vi "CloneClass.vi"(0 "ClassWriterNative.lvclass":refnum<class "ClassWriterNative.lvclass">, 1 "ClassRef":refnum<vi>, 2 "NewClassPath":path, 5 "error in (no error)":errorcluster) -> (14 "ClassWriterNative.lvclass":refnum<class "ClassWriterNative.lvclass">, 16 "NewClassPathOut(Might Be Modified)":path, 19 "error out":errorcluster)   [LabVIEW 2014, in "ClassWriterNative.lvclass"]
uses:
  <resource>/Framework/Providers/Open_GDS/ClassProviders/Provider_LvNativeClass/ClassWriterNative_class/ClassWriterNative.lvclass
  <vilib>/Utility/miscctls.llb/LVPointTypeDef.ctl
  <resource>/Framework/Providers/Open_GDS/ClassProviders/Common/ScriptingFunctions/Scripting.lvclass
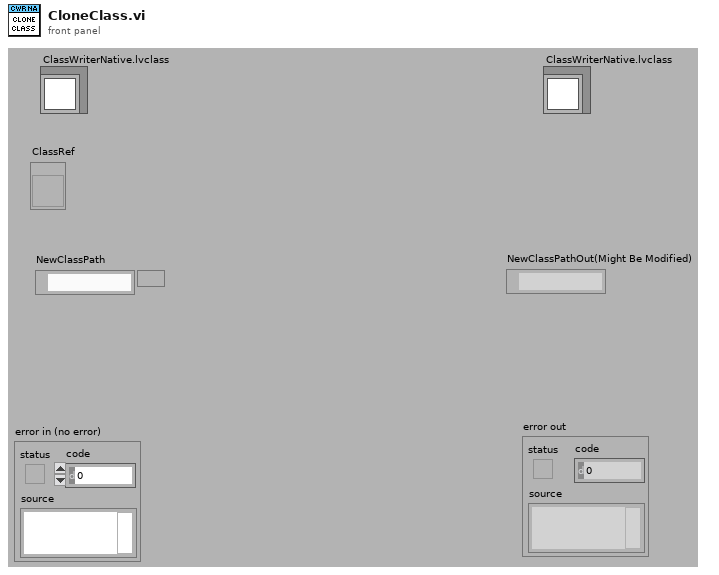
[diagram p1: front panel]
types:
  T1 = cluster{"NewClass":refnum<vi>, "OrgClassName":string, "NewClassName":string, "ProjectItemToAddTo":refnum<vi>, "Path":path, "Application":refnum<vi>, "VIRefs":refnum<vi>[]}
  T2 = typedef "LVPointTypeDef.ctl" = cluster{"Horizontal":i16, "Vertical":i16}
  T3 = enum32{"not a control VI", "control", "typedef", "strict typedef"}
  T4 = enum32{"invalid VI type", "Standard VI", "Control VI", "Global VI", "Polymorphic VI", "Configuration VI", "SubSystem", "Facade VI", "Method VI", "Statechart Diagram VI"}
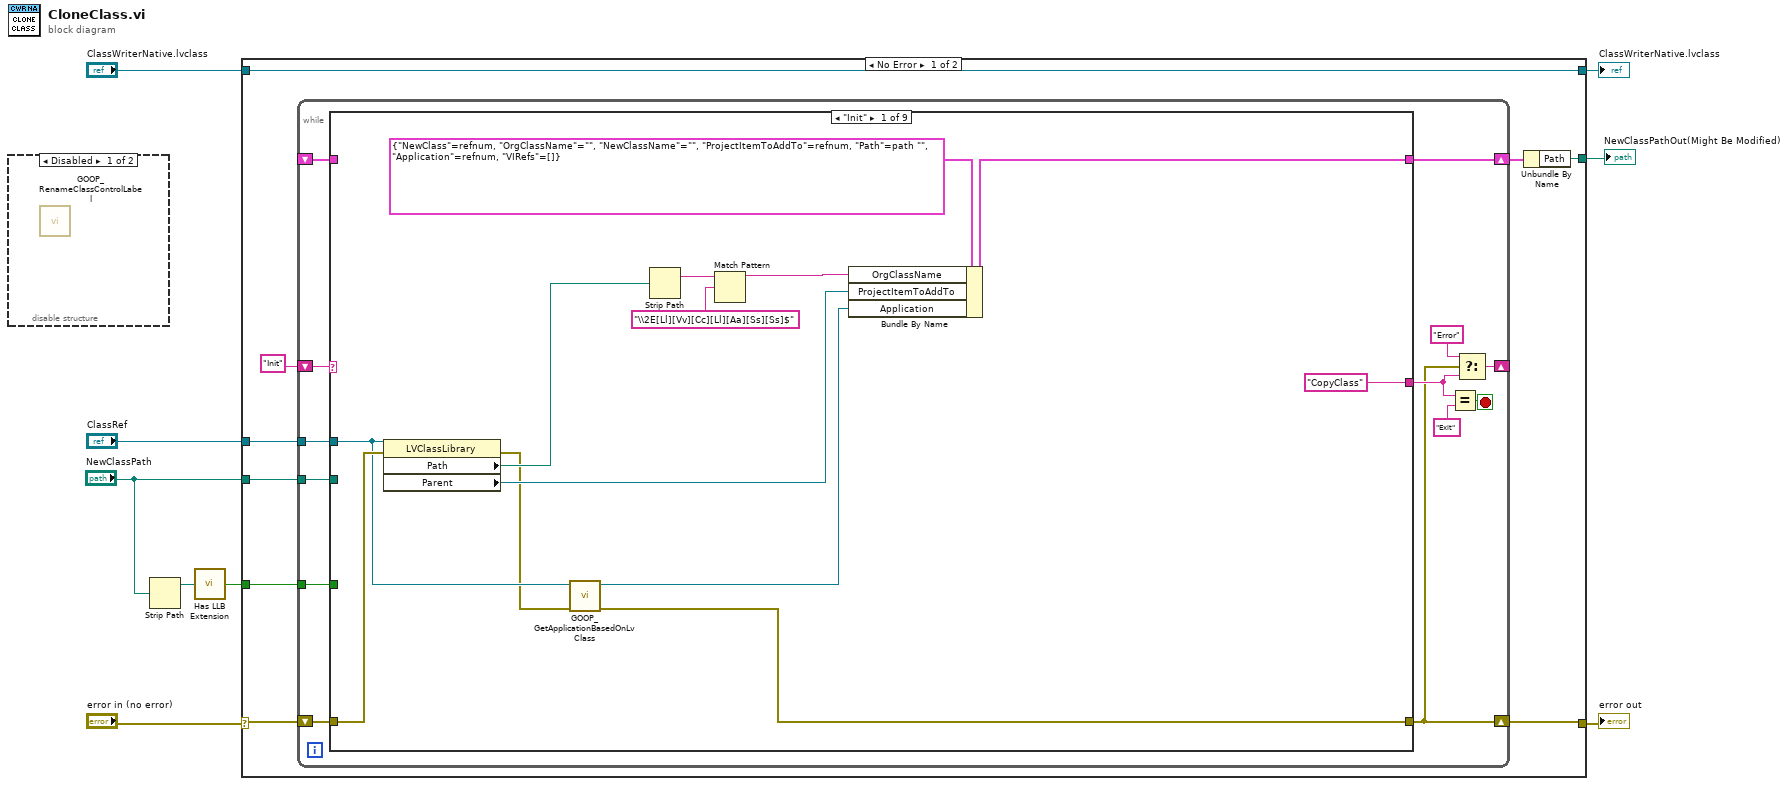
[diagram p0: block diagram]
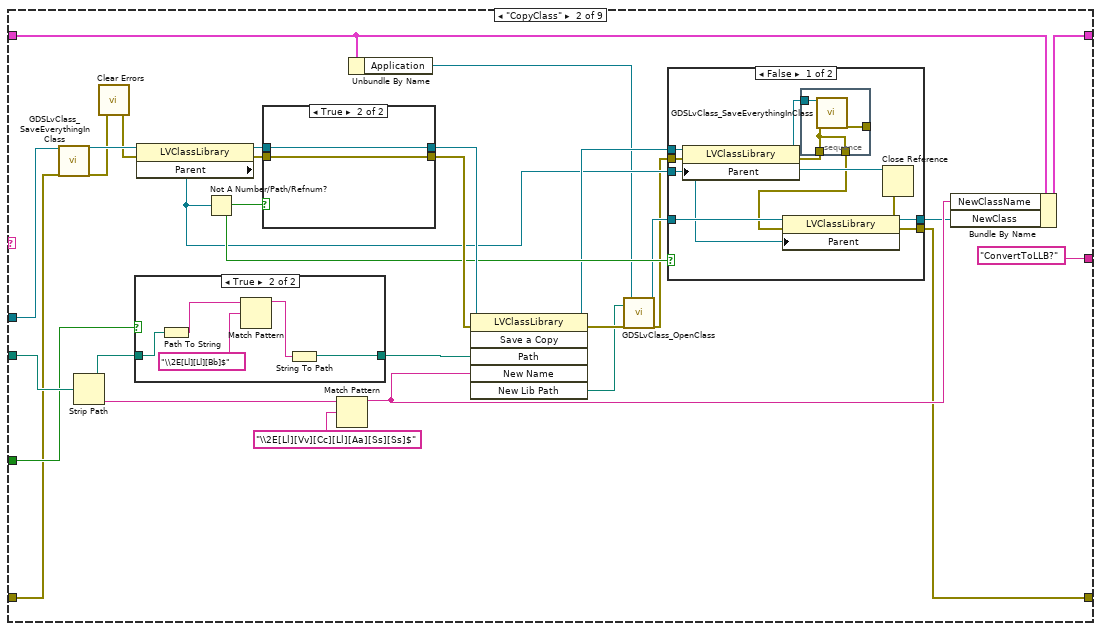
[diagram p3: hidden frame]
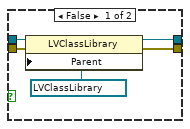
[diagram p6: hidden frame]
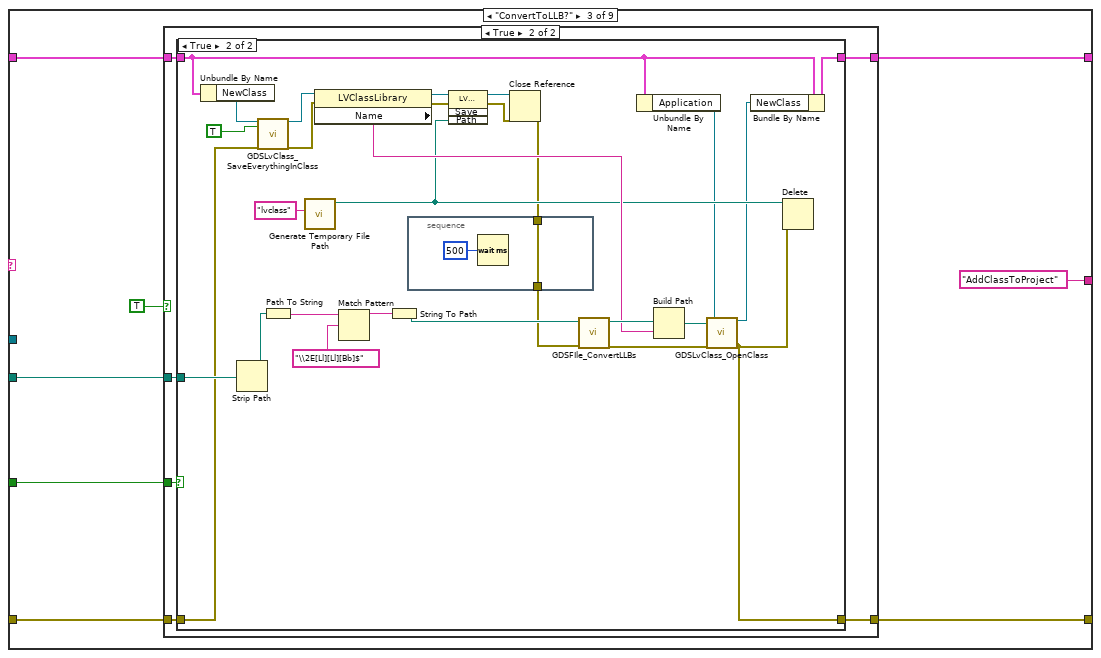
[diagram p7: hidden frame]
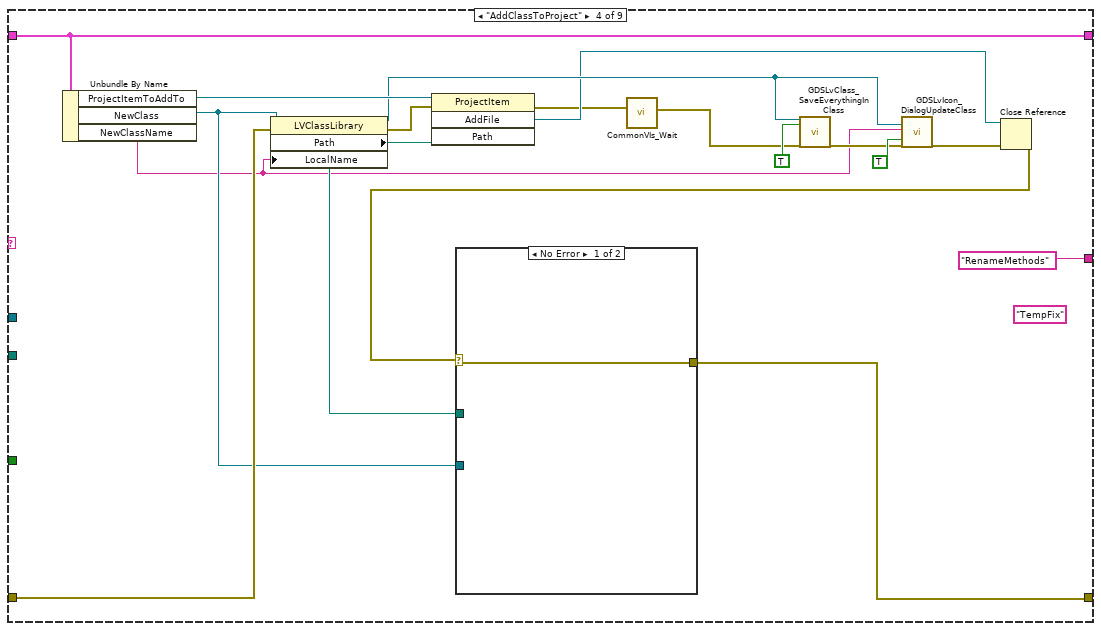
[diagram p10: hidden frame]
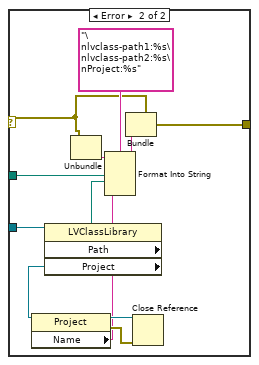
[diagram p11: hidden frame]
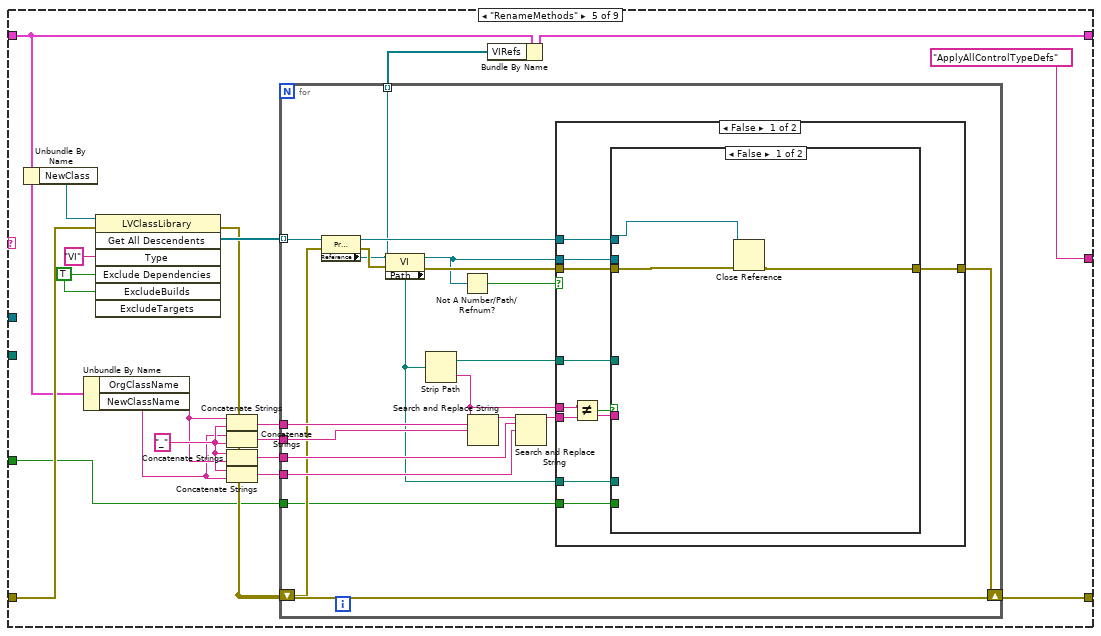
[diagram p12: hidden frame]
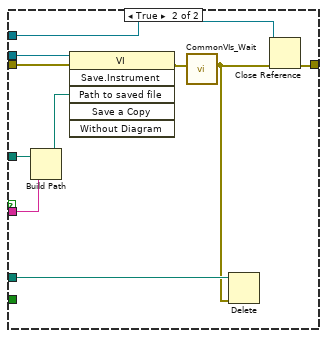
[diagram p13: hidden frame]
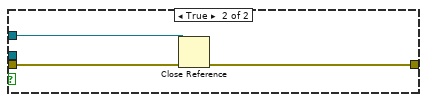
[diagram p14: hidden frame]
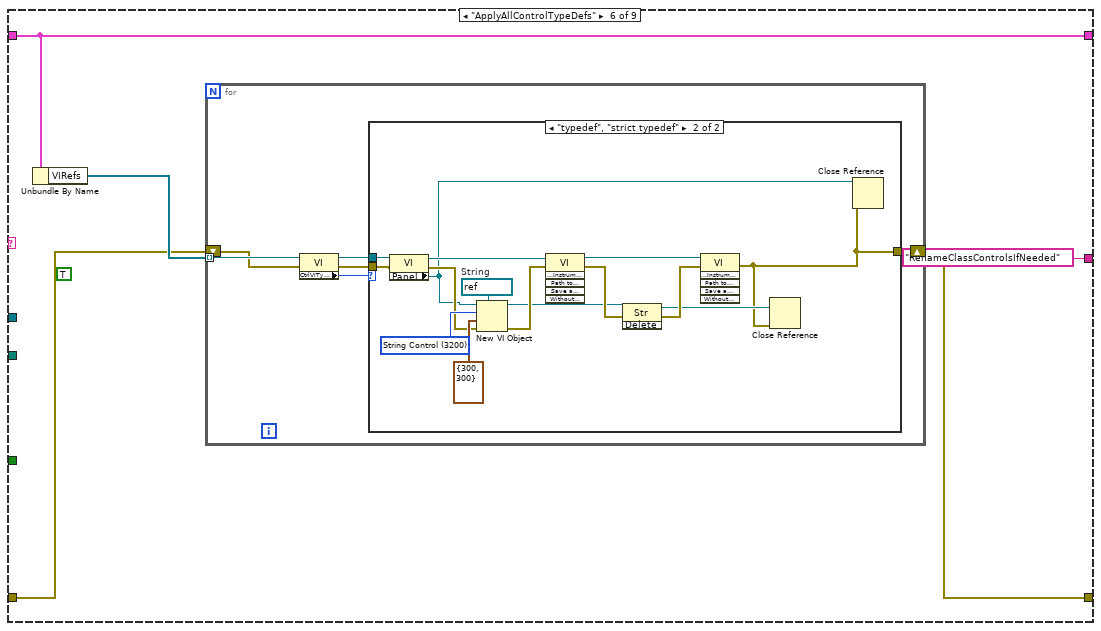
[diagram p15: hidden frame]
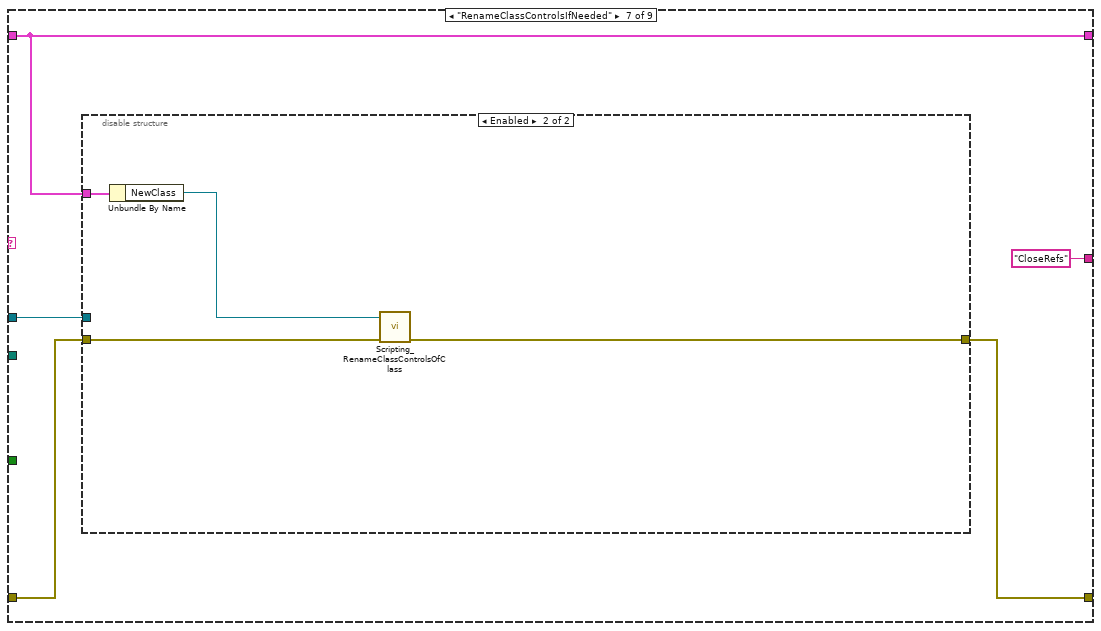
[diagram p17: hidden frame]
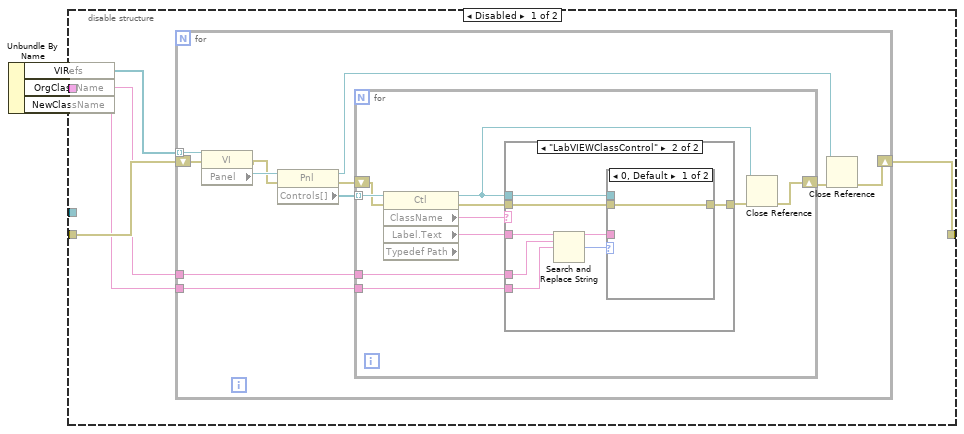
[diagram p18: hidden frame]
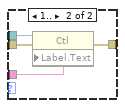
[diagram p20: hidden frame]
diagram:
  n1 = disable-structure shown="Disabled" {
    frame Disabled {
      n2 = call <resource>:"GOOP_RenameClassControlLabel.vi"() -> ()  [unwired: 10 in, 2 out]
    }
    frame Enabled {
    }
  }
  n3 = Strip Path(path="NewClassPath") -> (stripped path=w4:path)  [unwired: 1 out]
  n4 = call <vilib>:"Has LLB Extension.vi"("path"=w4) -> ("path to VI library?"=w2:bool)
  n5 = case shown="No Error" "error in (no error)" {
    selector: "error in (no error)" -> [w16 w385]
    tunnel: [w15 w385] -> w8
    tunnel: "ClassWriterNative.lvclass" -> [w18 w384]
    tunnel: [w18 w384] -> w6
    tunnel: "ClassRef" -> [w14 _]
    tunnel: "NewClassPath" -> [w13 _]
    tunnel: w2 -> [w12 _]
    tunnel: [w10 _] -> w1
    frame No Error {
      n6 = while {
        shift-right: [w24] -> w15
        shift-left: w16 -> [w31]
        shift-right: [w29] -> _
        shift-left: "Init" -> [w30]
        shift-right: [w23] -> w11
        shift-left: _ -> [w22]
        tunnel: w14 -> [w21]
        tunnel: w13 -> [w20]
        tunnel: w12 -> [w19]
        stop <- w28 stop-if-true
        n7 = case shown="\"Init\"" w30 {
          tunnel: w31 -> [w40 w49 w105 w162 w189 w243 w272 w321 w346]
          tunnel: [w32 w54 w104 w153 w186 w246 w273 w323 w345] -> w24
          tunnel: ["CopyClass" "ConvertToLLB?" "AddClassToProject" "RenameMethods" "ApplyAllControlTypeDefs" "RenameClassControlsIfNeeded" "CloseRefs" "Exit" "CloseRefs"] -> w25
          tunnel: [w38 w71 w101 w164 w181 w247 w274 w327 w347] -> w23
          tunnel: w22 -> [_ w46 w102 w164 w185 w247 w274 w328 w347]
          tunnel: w21 -> [w35 w67 _ _ _ _ w270 _ _]
          tunnel: w20 -> [_ w69 w107 _ _ _ _ _ _]
          tunnel: w19 -> [_ w50 w106 _ w183 _ _ _ _]
          frame "Init" {
            n8 = property class="LVClassLibrary"(reference=w35, error in=w40) -> (error out=w33:errorcluster, "Path"=w41:path, "Parent"=w36:refnum<vi>)  [unwired: 1 out]
            n9 = call <resource>:"GOOP_GetApplicationBasedOnLvClass.vi"("error in (no error)"=w33, "LVClassLibrary in"=w35) -> ("error out"=w32:errorcluster, "Application out"=w34:refnum<vi>)  [unwired: 8 in]
            n10 = Strip Path(path=w41) -> (name=w43:string)  [unwired: 1 out]
            n11 = Match Pattern(string=w43, regular expression="\\2E[Ll][Vv][Cc][Ll][Aa][Ss][Ss]$") -> (before substring=w37:string)  [unwired: 1 in, 3 out]
            n12 = Bundle By Name(cluster=T1 {"NewClass"=refnum, "OrgClassName"="", "NewClassName"="", "ProjectItemToAddTo"=refnum, "Path"=path "", "Application"=refnum, "VIRefs"=[]}, "OrgClassName"=w37, "ProjectItemToAddTo"=w36, "Application"=w34) -> (w38:T1)
          }
          frame "CopyClass" {
            n13 = call <resource>:"GDSLvClass_SaveEverythingInClass.vi"("ClassRefIn"=w67, "error in"=w49) -> ("ClassRefOut"=w64:refnum<vi>, "error out"=w48:errorcluster)  [unwired: 16 in]
            n14 = Strip Path(path=w69) -> (stripped path=w51:path, name=w73:string)
            n15 = call <vilib>:"Clear Errors.vi"("error in (no error)"=w48) -> ("error out"=w47:errorcluster)  [unwired: 5 in, 1 out]
            n16 = case shown="True" w50 {
              tunnel: w51 -> [w74 w79]
              tunnel: [w74 w78] -> w53
              frame False {
              }
              frame True {
                n17 = Path To String(path=w79) -> (string=w77:string)
                n18 = Match Pattern(string=w77, regular expression="\\2E[Ll][Ll][Bb]$") -> (before substring=w75:string)  [unwired: 1 in, 3 out]
                n19 = String To Path(string=w75) -> (path=w78:path)
              }
            }
            n20 = property class="LVClassLibrary"(reference=w64, error in=w47) -> (reference out=w66:refnum<vi>, error out=w63:errorcluster, "Parent"=w58:refnum<vi>)
            n21 = Not A Number/Path/Refnum?(number/path/refnum=w58) -> (NaN/Path/Refnum?=w60:bool)
            n22 = case shown="True" w60 {
              tunnel: w66 -> [w98 w100]
              tunnel: w63 -> [w96 w99]
              tunnel: [w95 w99] -> w62
              tunnel: [w94 w100] -> w61
              frame False {
                n23 = property class="LVClassLibrary"(reference=w98, error in=w96, "Parent"=refnum<vi> refnum ("Parent Class")) -> (reference out=w94:refnum<vi>, error out=w95:errorcluster)
              }
              frame True {
              }
            }
            n24 = Match Pattern(string=w73, regular expression="\\2E[Ll][Vv][Cc][Ll][Aa][Ss][Ss]$") -> (before substring=w65:string)  [unwired: 1 in, 3 out]
            n25 = Unbundle By Name(w46) -> ("Application"=w45:refnum<vi>)
            n26 = invoke class="LVClassLibrary" method="Save a Copy"(reference=w61, error in=w62, "Path"=w53, "New Name"=w65) -> (reference out=w59:refnum<vi>, error out=w70:errorcluster, "New Lib Path"=w68:path)  [unwired: 2 in, 3 out]
            n27 = call <resource>:"GDSLvClass_OpenClass.vi"("ClassToOpen"=w68, "error in (no error)"=w70, "Project/ApplicationRef(If empty, currect active project will be used)"=w45) -> ("LVClass.Open"=w57:refnum<vi>, "error out"=w55:errorcluster)  [unwired: 15 in]
            n28 = case shown="False" w60 {
              tunnel: w59 -> [w88 _]
              tunnel: w55 -> [w87 w92]
              tunnel: w58 -> [w83 _]
              tunnel: w57 -> [w86 w93]
              tunnel: [w85 w93] -> w56
              tunnel: [w84 w92] -> w54
              frame False {
                n29 = property class="LVClassLibrary"(reference=w88, error in=w87, "Parent"=w83) -> (reference out=w82:refnum<vi>, error out=w81:errorcluster)
                n30 = stacked-sequence {
                  tunnel: w82 -> [w91]
                  tunnel: w81 -> [w90]
                  tunnel: [w90] -> w80
                  tunnel: [w89] -> _
                  frame #0 {
                    n31 = call <resource>:"GDSLvClass_SaveEverythingInClass.vi"("ClassRefIn"=w91, "error in"=w90) -> ("error out"=w89:errorcluster)  [unwired: 16 in, 1 out]
                  }
                }
                n32 = property class="LVClassLibrary"(reference=w86, error in=w80, "Parent"=w83) -> (reference out=w85:refnum<vi>, error out=w84:errorcluster)
                n33 = Close Reference(reference=w83, error in (no error)=w84) -> ()  [unwired: 1 out]
              }
              frame True {
              }
            }
            n34 = Bundle By Name(cluster=w46, "NewClassName"=w65, "NewClass"=w56) -> (w71:T1)
          }
          frame "ConvertToLLB?" {
            n35 = case shown="True" TRUE {
              tunnel: w107 -> [_ w116]
              tunnel: w106 -> [_ w115]
              tunnel: w105 -> [w110 w114]
              tunnel: [w110 w113] -> w104
              tunnel: w102 -> [w109 w112]
              tunnel: [w109 w111] -> w101
              frame False {
              }
              frame True {
                n36 = case shown="True" w115 {
                  tunnel: w116 -> [_ w143]
                  tunnel: w114 -> [w118 w134]
                  tunnel: [w118 w123] -> w113
                  tunnel: w112 -> [w117 w122]
                  tunnel: [w117 w140] -> w111
                  frame False {
                  }
                  frame True {
                    n37 = Unbundle By Name(w122) -> ("NewClass"=w136:refnum<vi>)
                    n38 = Strip Path(path=w143) -> (stripped path=w142:path)  [unwired: 1 out]
                    n39 = call <resource>:"GDSLvClass_SaveEverythingInClass.vi"("ClassRefIn"=w136, "ForceResaving(False)"=TRUE, "error in"=w134) -> ("ClassRefOut"=w135:refnum<vi>, "error out"=w133:errorcluster)  [unwired: 15 in]
                    n40 = Path To String(path=w142) -> (string=w146:string)
                    n41 = call <vilib>:"Generate Temporary File Path.vi"("Temporary File Extension (tmp)"="lvclass") -> ("Unique Temporary File Path"=w127:path)  [unwired: 9 in, 1 out]
                    n42 = property class="LVClassLibrary"(reference=w135, error in=w133) -> (reference out=w130:refnum<vi>, error out=w129:errorcluster, "Name"=w138:string)
                    n43 = Match Pattern(string=w146, regular expression="\\2E[Ll][Ll][Bb]$") -> (before substring=w144:string)  [unwired: 1 in, 3 out]
                    n44 = String To Path(string=w144) -> (path=w141:path)
                    n45 = invoke class="LVClassLibrary" method="Save"(reference=w130, error in=w129, "Path"=w127) -> (reference out=w125:refnum<vi>, error out=w124:errorcluster)  [unwired: 1 in, 2 out]
                    n46 = Close Reference(reference=w125, error in (no error)=w124) -> (error out=w120:errorcluster)
                    n47 = stacked-sequence {
                      tunnel: w120 -> [w148]
                      tunnel: [w148] -> w119
                      frame #0 {
                        n48 = Wait (ms)(milliseconds to wait=u32 500) -> ()  [unwired: 1 out]
                      }
                    }
                    n49 = call <resource>:"GDSFIle_ConvertLLBs.vi"("error in (no error)"=w119, "ClassPath Or LLB Path"=w141) -> ("error out"=w132:errorcluster, "ClassPath Or LLB Path Out"=w139:path)  [unwired: 8 in]
                    n50 = Unbundle By Name(w122) -> ("Application"=w121:refnum<vi>)
                    n51 = Build Path(base path=w139, name or relative path=w138) -> (appended path=w131:path)
                    n52 = call <resource>:"GDSLvClass_OpenClass.vi"("ClassToOpen"=w131, "error in (no error)"=w132, "Project/ApplicationRef(If empty, currect active project will be used)"=w121) -> ("LVClass.Open"=w126:refnum<vi>, "error out"=w123:errorcluster)  [unwired: 15 in]
                    n53 = Bundle By Name(cluster=w122, "NewClass"=w126) -> (w140:T1)
                    n54 = Delete(path (use dialog)=w127, error in=w123) -> ()  [unwired: 3 in, 3 out]
                  }
                }
              }
            }
          }
          frame "AddClassToProject" {
            (unwired) "TempFix"
            n55 = Unbundle By Name(w164) -> ("ProjectItemToAddTo"=w166:refnum<vi>, "NewClass"=w158:refnum<vi>, "NewClassName"=w149:string)
            n56 = property class="LVClassLibrary"(reference=w158, error in=w162, "LocalName"=w149) -> (reference out=w160:refnum<vi>, error out=w165:errorcluster, "Path"=w157:path)
            n57 = invoke class="ProjectItem" method="AddFile"(reference=w166, error in=w165, "Path"=w157) -> (error out=w151:errorcluster, "AddFile"=w156:refnum<vi>)  [unwired: 1 in, 2 out]
            n58 = call <resource>:"CommonVIs_Wait.vi"("error in"=w151) -> ("error out"=w150:errorcluster)  [unwired: 9 in]
            n59 = call <resource>:"GDSLvClass_SaveEverythingInClass.vi"("ClassRefIn"=w160, "ForceResaving(False)"=TRUE, "error in"=w150) -> ("error out"=w159:errorcluster)  [unwired: 15 in, 1 out]
            n60 = call <resource>:"GDSLvIcon_DialogUpdateClass.vi"("ClassPath(FilePath/ProjectTreePath/LvCLassRef)"=w160, "ClassName"=w149, "AutoUpdate"=TRUE, "error in (no error)"=w159) -> ("error out"=w155:errorcluster)  [unwired: 12 in, 3 out]
            n61 = Close Reference(reference=w156, error in (no error)=w155) -> (error out=w154:errorcluster)
            n62 = case shown="No Error" w154 {
              selector: w154 -> [w167 w168]
              tunnel: w158 -> [_ w173]
              tunnel: w157 -> [_ w172]
              tunnel: [w167 w171] -> w153
              frame No Error {
              }
              frame Error {
                n63 = property class="LVClassLibrary"(reference=w173) -> ("Path"=w178:path, "Project"=w177:refnum<vi>)  [unwired: 1 in, 2 out]
                n64 = property class="Project"(reference=w177) -> (reference out=w176:refnum<vi>, error out=w175:errorcluster, "Name"=w174:string)  [unwired: 1 in]
                n65 = Unbundle(w168) -> ("source"=w170:string)  [unwired: 2 out]
                n66 = Format Into String(format string="\nlvclass-path1:%s\nlvclass-path2:%s\nProject:%s", initial string=w170, w172, w178, w174) -> (resulting string=w169:string)  [unwired: 1 in, 1 out]
                n67 = Bundle(cluster=w168, "source"=w169) -> (w171:errorcluster)  [unwired: 2 in]
                n68 = Close Reference(reference=w176, error in (no error)=w175) -> ()  [unwired: 1 out]
              }
            }
          }
          frame "RenameMethods" {
            w184 = TRUE ("ExcludeDependencies")
            w193 = "_" ("string")
            n69 = Unbundle By Name(w185) -> ("NewClass"=w197:refnum<vi>)
            n70 = Unbundle By Name(w185) -> ("OrgClassName"=w188:string, "NewClassName"=w187:string)
            n71 = invoke class="LVClassLibrary" method="Get All Descendents"(reference=w197, error in=w189, "Type"="VI", "Exclude Dependencies"=w184, "ExcludeBuilds"=w184) -> (error out=w186:errorcluster, "All Descendents"=w190:refnum<vi>[])  [unwired: 2 in, 5 out]
            n72 = Concatenate Strings(w188, w193) -> (w192:string)
            n73 = Concatenate Strings(w187, w193) -> (w191:string)
            n74 = Concatenate Strings(w193, w188) -> (w194:string)
            n75 = Concatenate Strings(w193, w187) -> (w195:string)
            n76 = for {
              tunnel: w190 -> [w205] mode=indexing
              tunnel: w192 -> [w216]
              tunnel: w191 -> [w215]
              tunnel: w194 -> [w212]
              tunnel: w195 -> [w211]
              shift-right: [w201] -> _
              shift-left: w186 -> [w210]
              tunnel: w183 -> [w199]
              tunnel: [w198] -> w180 mode=indexing
              n77 = property class="ProjectItem"(reference=w205, error in=w210) -> (reference out=w204:refnum<vi>, error out=w209:errorcluster, "Reference"=w198:refnum<vi>)
              n78 = property class="VI"(reference=w198, error in=w209) -> (reference out=w200:refnum<vi>, error out=w202:errorcluster, "Path"=w203:path)
              n79 = Strip Path(path=w203) -> (stripped path=w206:path, name=w207:string)
              n80 = Not A Number/Path/Refnum?(number/path/refnum=w200) -> (NaN/Path/Refnum?=w214:bool)
              n81 = Search and Replace String(input string=w207, search string=w216, replace string=w215) -> (result string=w213:string)  [unwired: 5 in, 3 out]
              n82 = Search and Replace String(input string=w213, search string=w212, replace string=w211) -> (result string=w208:string)  [unwired: 5 in, 3 out]
              n83 = case shown="False" w214 {
                tunnel: w200 -> [w226 _]
                tunnel: w208 -> [w223 _]
                tunnel: w207 -> [w225 _]
                tunnel: w206 -> [w222 _]
                tunnel: w204 -> [w221 w242]
                tunnel: w203 -> [w220 _]
                tunnel: w202 -> [w219 w241]
                tunnel: [w218 w240] -> w201
                tunnel: w199 -> [w217 _]
                frame False {
                  n84 = Not Equal?(x=w225, y=w223) -> (x != y?=w224:bool)
                  n85 = case shown="False" w224 {
                    tunnel: w226 -> [_ w236]
                    tunnel: w223 -> [_ w239]
                    tunnel: w222 -> [_ w238]
                    tunnel: w221 -> [w228 w233]
                    tunnel: w220 -> [_ w235]
                    tunnel: w219 -> [w227 w234]
                    tunnel: [w229 w232] -> w218
                    tunnel: w217 -> [_ _]
                    frame False {
                      n86 = Close Reference(reference=w228, error in (no error)=w227) -> (error out=w229:errorcluster)
                    }
                    frame True {
                      n87 = Build Path(base path=w238, name or relative path=w239) -> (appended path=w237:path)
                      n88 = invoke class="VI" method="Save.Instrument"(reference=w236, error in=w234, "Path to saved file"=w237) -> (error out=w231:errorcluster)  [unwired: 3 in, 5 out]
                      n89 = call <resource>:"CommonVIs_Wait.vi"("error in"=w231) -> ("error out"=w230:errorcluster)  [unwired: 9 in]
                      n90 = Delete(path (use dialog)=w235, error in=w230) -> ()  [unwired: 3 in, 3 out]
                      n91 = Close Reference(reference=w233, error in (no error)=w230) -> (error out=w232:errorcluster)
                    }
                  }
                }
                frame True {
                  n92 = Close Reference(reference=w242, error in (no error)=w241) -> (error out=w240:errorcluster)
                }
              }
            }
            n93 = Bundle By Name(cluster=w185, "VIRefs"=w180) -> (w181:T1)
          }
          frame "ApplyAllControlTypeDefs" {
            (unwired) TRUE ("ExcludeDependencies")
            n94 = Unbundle By Name(w247) -> ("VIRefs"=w244:refnum<vi>[])
            n95 = for {
              shift-right: [w252] -> w246
              shift-left: w243 -> [w248]
              tunnel: w244 -> [w249] mode=indexing
              n96 = property class="VI"(reference=w249, error in=w248) -> (reference out=w251:refnum<vi>, error out=w253:errorcluster, "CtrlVIType"=w250:T3)
              n97 = case shown="\"typedef\", \"strict typedef\"" w250 {
                tunnel: w251 -> [_ w267]
                tunnel: w253 -> [w254 w264]
                tunnel: [w254 w255] -> w252
                frame Default {
                }
                frame "typedef", "strict typedef" {
                  w268 = refnum<vi> refnum  # String
                  w269 = 3200 items=[".NET Refnum"=3441, "Absolute Value"=1054, "Access Rights"=1412, "ActiveX Container"=2072, "Add"=1050, "Add Array Elements"=1903, "Agitator"=3831, "AllSpoll"=1960, "And"=1061, "And Array Elements"=1911, "Append True/False String"=1511, "Application Refnum"=3412, "Array"=3300, "Array 1"=21608, "Array Constant"=2070, "Array Max & Min"=1907, "Array Size"=1809, "Array Subset"=2044, "Array To Cluster"=1168, "Array To Spreadsheet String"=1540, "Array of Strings to Path"=1422, "Atmospheric Tank"=3070, "Atmospheric Tank 1"=21751, "Automation Close"=8001, "Automation Open"=8000, "Automation Refnum"=3410, "Avogadro Constant (1/mol)"=2030, "Base 10 Logarithm Of e"=2022, "Bin"=3073, "Bin 1"=21755, "Boolean Array To Number"=1815, "Boolean To (0,1)"=1167, "Build Array"=2041, "Build Cluster Array"=2047, "Build Path"=1419, "Build Waveform"=2066, "Bundle"=2049, "Bundle By Name"=2057, "Byte Array To String"=1609, "Byte Stream File Refnum"=3408, "Call By Reference Node"=3901, "Call Chain"=1999, "Call Library Function Node"=2062, "Cancel Button"=3131, "Cancel Button 1"=21739, "Cancel Notification"=9107, "Carriage Return Constant"=2010, "Case Structure"=2001, "Cast Unit Bases"=1079, "Check Valve"=3833, "Checkbox"=3117, "Class Specifier Constant"=2094, "Close File"=1405, "Close Reference"=8011, "Cluster"=3400, "Cluster 1"=21607, "Cluster Constant"=2071, "Cluster To Array"=1169, "Code Interface Node"=2050, "Color Box"=3013, "Color Box Constant"=2120, "Color Box Thin Border"=2905, "Color Ramp"=3022, "Combo Box"=21604, "Combo Box 1"=3304, "Combo Box Constant"=2088, "Complex Conjugate"=1048, "Complex To Polar"=1045, "Complex To Re/Im"=1044, "Compound Arithmetic"=2200, "Compressor"=3832, "Concatenate Strings"=2040, "Conditional Disable Structure"=2064, "Constructor Node"=3904, "Control Help Window"=1353, "Control Online Help"=1355, "Control Refnum"=3419, "Convert Unit"=2059, "Conveyer"=3827, "Copy"=1416, "Cosecant"=1204, "Cosine"=1201, "Cotangent"=1205, "Create User Event"=2073, "Current VI's Menubar"=9000, "Current VI's Path"=1426, "DAQmx Analog Trigger Source"=3336, "DAQmx Analog Trigger Source 1"=21774, "DAQmx Analog Trigger Source 2"=21951, "DAQmx Analog Trigger Source Constant"=2119, "DAQmx Device Name"=3318, "DAQmx Device Name 1"=21950, "DAQmx Device Name 2"=21773, "DAQmx Device Name Constant"=2093, "DAQmx Global Channel"=3443, "DAQmx Global Channel 1"=21770, "DAQmx Global Channel 2"=21957, "DAQmx Global Channel Constant"=3430, "DAQmx Physical Channel"=21777, "DAQmx Physical Channel 1"=21954, "DAQmx Physical Channel 2"=3335, "DAQmx Physical Channel Constant"=2118, "DAQmx Scale Name"=21952, "DAQmx Scale Name 1"=21775, "DAQmx Scale Name 2"=3317, "DAQmx Scale Name Constant"=2116, "DAQmx Switch"=21953, "DAQmx Switch 1"=3337, "DAQmx Switch 2"=21776, "DAQmx Switch Constant"=2121, "DAQmx Task Name"=3442, "DAQmx Task Name 1"=21778, "DAQmx Task Name 2"=21959, "DAQmx Task Name Constant"=3434, "DAQmx Terminal"=21955, "DAQmx Terminal 1"=21781, "DAQmx Terminal 2"=3319, "DAQmx Terminal Constant"=2117, "Data Log File Refnum"=3402, "DataSocket Close"=1085, "DataSocket Open"=1084, "DataSocket Read"=1086, "DataSocket Refnum"=3417, "DataSocket Write"=1087, "Database Variant To Data"=8004, "Date/Time To Seconds"=1308, "Decimal Digit?"=1119, "Decimal String To Number"=1184, "Decimate 1D Array"=2046, "Decrement"=1058, "Default Directory"=1427, "Delete"=1417, "Delete From Array"=3912, "Delete Menu Items"=9004, "Delete Variant Attribute"=8206, "Delete Waveform Attribute"=8209, "Dequeue Element"=9113, "Destroy User Event"=2075, "DevClear"=1961, "DevClearList"=1962, "Device Control/Status"=1433, "Device Refnum"=3405, "Diagram Disable Structure"=2054, "Dial"=21732, "Dial 1"=3050, "Dialog Button"=3130, "Dialog Checkbox"=3132, "Dialog Chiseled Line"=3632, "Dialog Colored Rectangle"=3625, "Dialog Combo Box"=21917, "Dialog Horizontal Pointer Slide"=21902, "Dialog Horizontal Progress Bar"=21910, "Dialog Horizontal Slide"=21904, "Dialog Label"=21961, "Dialog Listbox"=2105, "Dialog Listbox 1"=21921, "Dialog Multicolumn Listbox"=21220, "Dialog Multiple Selection Multicolumn Listbox"=21221, "Dialog Numeric"=21919, "Dialog Path Control"=21922, "Dialog Pict Ring"=21925, "Dialog Radio Button"=3133, "Dialog Recessed Frame"=3624, "Dialog Ring"=3060, "Dialog Spin Control"=21900, "Dialog String"=21920, "Dialog Tab Control"=3331, "Dialog Table"=21225, "Dialog Tree"=21794, "Dialog Vertical Pointer Slide"=21901, "Dialog Vertical Progress Bar"=21909, "Dialog Vertical Slide"=21903, "Digital Data"=3210, "Digital Data 1"=21216, "Digital Waveform Graph"=3511, "Digital Waveform Graph 1"=21718, "Digital Waveform Graph 2"=3502, "Divide"=1053, "Dlg CheckBox"=21924, "Dlg Horiz Scrollbar"=21905, "Dlg Numeric"=2100, "Dlg Numeric 2"=3006, "Dlg String"=2110, "Dlg Vert Scrollbar"=21906, "Down Arrow"=3824, "Down Bow Valve"=3707, "Down Bow Valve 1"=21767, "Down Bow Valve 2"=3807, "Down Rect Valve"=21766, "Down Rect Valve 1"=3706, "Down Rect Valve 2"=3806, "Down Tee"=3818, "Down Tee 1"=3718, "EOF"=1410, "Elementary Charge (C)"=2027, "Empty Path Constant"=2033, "Empty String Constant"=2013, "Empty String/Path?"=1112, "Enable Menu Tracking"=9002, "EnableLocal"=1963, "EnableRemote"=1964, "End of Line Constant"=2035, "Enqueue Element"=9111, "Enqueue Element At Opposite End"=9129, "Enum"=21605, "Enum 1"=3023, "Enum Constant"=2090, "Equal To 0?"=1113, "Equal?"=1102, "Error Ring Constant"=2039, "Event Callback Refnum"=3435, "Event Structure"=2052, "Exchanger"=3828, "Exclusive Or"=1063, "Exponential"=1211, "Exponential (Arg) -1"=1222, "Expression Node"=2201, "False Constant"=2006, "Feedback Node"=2353, "FieldPoint IO Point"=3439, "FieldPoint IO Point 1"=21784, "FieldPoint IO Point Constant"=3440, "File Dialog"=8081, "File Path Control"=21730, "File Path Control 1"=3203, "File Path Indicator"=21731, "File Path Indicator 1"=3204, "File/Directory Info"=1413, "FindLstn"=1965, "FindRQS"=1966, "First Call?"=1083, "Flat Box"=3602, "Flat Circle"=3605, "Flat Down Triangle"=3623, "Flat Frame"=3608, "Flat Left Triangle"=3620, "Flat Right Triangle"=3621, "Flat Round Button"=3102, "Flat Rounded Box"=3611, "Flat Sequence Structure"=2069, "Flat Square Button"=3103, "Flat Up Triangle"=3622, "Flatten To String"=1160, "Flatten To XML"=8400, "Flattened String To Variant"=8202, "Flush File"=1406, "Flush Queue"=9114, "For Loop"=2002, "Format Date/Time String"=8100, "Format Into File"=2083, "Format Into String"=2081, "Format Value"=1512, "Formula Node"=2004, "Fract/Exp String To Number"=1187, "Framed Color Box"=21019, "Framed Color Box 1"=3008, "Free Label"=2321, "Furnace"=3829, "GPIB Clear"=1954, "GPIB Initialization"=1957, "GPIB Misc"=1956, "GPIB Read"=1951, "GPIB Serial Poll"=1955, "GPIB Status"=1959, "GPIB Trigger"=1953, "GPIB Wait"=1958, "GPIB Write"=1950, "Gauge"=21009, "Gauge 1"=3040, "Generate Front Panel Activity"=1329, "Generate Occurrence"=1700, "Generate User Event"=2074, "Generic Refnum"=3428, "Generic Refnum By Reference Flatten"=3453, "Generic Refnum Deep Copy"=3447, "Generic Refnum Name"=21745, "Generic Refnum Tag"=3429, "Generic Refnum Tag By Reference Flatten"=3454, "Generic Refnum Tag Flatten"=21747, "Get Date/Time In Seconds"=1303, "Get Date/Time String"=1600, "Get Help Window Status"=1354, "Get Menu Item Info"=9005, "Get Menu Selection"=9001, "Get Menu Short Cut Info"=9007, "Get Notifier Status"=9103, "Get Queue Status"=9110, "Get Variant Attribute"=8205, "Get Waveform Attribute"=8208, "Get Waveform Components"=2067, "Global Variable"=2060, "Gravitational Constant (N m2/kg2)"=2029, "Greater Or Equal To 0?"=1114, "Greater Or Equal?"=1103, "Greater Than 0?"=1117, "Greater?"=1110, "Handle Peek"=1604, "Handle Poke"=1605, "Hex Digit?"=1123, "Hexadecimal String To Number"=1185, "HiQ-Script"=9021, "Hopper"=3072, "Hopper 1"=21754, "Horiz Line"=3821, "Horiz Pipe"=3810, "Horiz Pipe 1"=3710, "Horizontal Button Box"=3636, "Horizontal Fill Slide"=21100, "Horizontal Fill Slide 1"=3012, "Horizontal Graduated Bar"=21106, "Horizontal Pointer Slide"=3011, "Horizontal Pointer Slide 1"=21101, "Horizontal Progress Bar"=21102, "Horizontal Slide"=3010, "Horizontal Slide Switch"=3114, "Horizontal Smooth Box"=3633, "Horizontal Switch"=3108, "Horizontal Tank"=3071, "Horizontal Toggle Switch"=3110, "Horizontal Toggle Switch 1"=21700, "Hyperbolic Cosine"=1215, "Hyperbolic Sine"=1214, "Hyperbolic Tangent"=1216, "IMAQ Session"=3415, "IP To String"=1710, "IVI Delete Session"=8103, "IVI Logical Name"=3414, "IVI Logical Name 1"=21736, "IVI Logical Name Constant"=3420, "IVI New Session"=8102, "Implies"=1080, "In Range and Coerce"=1127, "Increment"=1057, "Index & Bundle Cluster Array"=2056, "Index Array"=2042, "Index String Array"=1531, "Initialize Array"=2053, "Insert Into Array"=3911, "Insert Menu Items"=9003, "Intensity Chart"=3509, "Intensity Chart 1"=21719, "Intensity Graph"=3510, "Intensity Graph 1"=21720, "Interleave 1D Arrays"=2045, "Interpolate 1D Array"=1905, "Inverse Cosine"=1207, "Inverse Hyperbolic Cosine"=1218, "Inverse Hyperbolic Sine"=1217, "Inverse Hyperbolic Tangent"=1219, "Inverse Sine"=1206, "Inverse Tangent"=1208, "Inverse Tangent (2 Input)"=1228, "Invoke Node"=3900, "IrDA Close Connection"=9144, "IrDA Create Listener"=9140, "IrDA Discover"=9141, "IrDA Network Connection Refnum"=3450, "IrDA Open Connection"=9142, "IrDA Read"=9145, "IrDA Wait On Listener"=9143, "IrDA Write"=9146, "Join Numbers"=1171, "Knob"=21000, "Knob 1"=3005, "LED Button"=3116, "Label"=21960, "Labeled Oblong Button"=3125, "Labeled Rectangular Button"=3124, "Labeled Round Button"=3122, "Labeled Square Button"=3123, "Left Arrow"=3826, "Left Bow Valve"=3701, "Left Bow Valve 1"=21761, "Left Bow Valve 2"=3801, "Left Down Elbow"=3711, "Left Down Elbow 1"=3811, "Left Pump"=3713, "Left Pump 1"=3813, "Left Rect Valve"=21760, "Left Rect Valve 1"=3700, "Left Rect Valve 2"=3800, "Left Tee"=3709, "Left Tee 1"=3809, "Left Up Elbow"=3808, "Left Up Elbow 1"=3708, "Less Or Equal To 0?"=1115, "Less Or Equal?"=1104, "Less Than 0?"=1118, "Less?"=1111, "Lexical Class"=1126, "Line Feed Constant"=2011, "List Directory"=1418, "Listbox"=21210, "Listbox 1"=3206, "Listbox Symbol Ring Constant"=2038, "Local Variable"=2061, "Lock Range"=1411, "Logarithm Base 10"=1210, "Logarithm Base 2"=1225, "Logarithm Base X"=1224, "Logical Shift"=1081, "Lowered Rounded Box"=3638, "MATLAB Script"=9020, "MakeAddr"=1967, "Mantissa & Exponent"=1150, "Match First String"=1532, "Match Pattern"=1535, "Match True/False String"=1533, "Max & Min"=1108, "Menu Refnum"=3413, "Menu Ring"=3018, "Menu Ring 1"=21600, "Menu-Popup Ring"=3017, "Merge Signals"=2350, "Meter"=21008, "Meter 1"=3030, "Molar Gas Constant (J/(mol K))"=2032, "Motion Resource"=3448, "Motion Resource 1"=21787, "Motion Resource Constant"=3449, "Motor"=3820, "Motor 1"=3720, "Move"=1415, "Multicolumn Listbox"=21214, "Multicolumn Listbox 1"=21215, "Multicolumn Listbox 2"=21204, "Multicolumn Listbox 3"=21205, "Multicolumn Listbox 4"=3307, "Multiple Selection Listbox"=3208, "Multiple Selection Listbox 1"=21201, "Multiple Selection Listbox 2"=21211, "Multiple Selection Listbox 3"=3207, "Multiple Selection Multicolumn Listbox"=3308, "Multiply"=1052, "Multiply Array Elements"=1904, "Natural Logarithm"=1209, "Natural Logarithm (Arg +1)"=1221, "Natural Logarithm Base"=2020, "Natural Logarithm Of 10"=2023, "Natural Logarithm Of 2"=2024, "Natural Logarithm Of Pi"=2018, "Negate"=1069, "Negative Infinity"=2019, "New Directory"=1402, "New File"=1404, "New VI"=8014, "New VI Object"=8015, "Not"=1064, "Not A Number/Path/Refnum?"=1128, "Not A Path Constant"=2034, "Not And"=1071, "Not Equal To 0?"=1116, "Not Equal?"=1105, "Not Exclusive Or"=1073, "Not Or"=1072, "Not a Refnum Constant"=2036, "Not a Tag"=2037, "Number To Boolean Array"=1814, "Number To Decimal String"=1180, "Number To Engineering String"=1183, "Number To Exponential String"=1505, "Number To Fractional String"=1506, "Number To Hexadecimal String"=1181, "Number To Octal String"=1182, "Numeric Constant"=2005, "Numeric Control"=21003, "Numeric Control 1"=3000, "Numeric Indicator"=21004, "Numeric Indicator 1"=3001, "OK Button"=21738, "OLE Variant"=3150, "Obtain Notifier"=9101, "Obtain Queue"=9108, "Occurrence Refnum"=3406, "Octal Digit?"=1129, "Octal String To Number"=1186, "Old VISA Open"=1921, "One Button Dialog"=1340, "Open Application Reference"=8012, "Open Device"=1430, "Open File"=1403, "Open File (New)"=8050, "Open Tank"=21752, "Open Tank 1"=3074, "Open VI Object Reference"=8013, "Open VI Reference"=8010, "Or"=1062, "Or Array Elements"=1910, "PPoll"=1969, "PPollConfig"=1970, "PPollUnconfig"=1971, "PassControl"=1968, "Path Constant"=2009, "Path To String"=1077, "Path Type"=1421, "Path to Array of Strings"=1423, "Pi"=2014, "Pi Divided By 2"=2016, "Pi Multiplied By 2"=2015, "Pick Line"=1510, "Pict Ring"=21602, "Pict Ring 1"=3015, "Picture"=3508, "PixMap"=3505, "PixMap (Do not touch it!!)"=3507, "Planck Constant (J/Hz)"=2026, "Platform Flat Square Button"=3134, "Plug-In Control"=21820, "Polar To Complex"=1047, "Positive Infinity"=2025, "Power Of 10"=1212, "Power Of 2"=1223, "Power Of X"=1213, "Pressure Tank"=3075, "Pressure Tank 1"=21753, "Preview Queue Element"=9112, "Printable?"=1124, "Property Node"=1920, "Pulldown Menu Ring"=3061, "Push Button"=21001, "Quit LabVIEW"=1352, "Quotient & Remainder"=1056, "Raised Box"=3637, "Raised Box 1"=3600, "Raised Circle"=3603, "Raised Down Triangle"=3615, "Raised Frame"=3606, "Raised Left Triangle"=3612, "Raised Right Triangle"=3613, "Raised Rounded Box"=3609, "Raised Up Triangle"=3614, "Random Number (0-1)"=1070, "RcvRespMsg"=1972, "Re/Im To Complex"=1046, "Read Binary File"=8051, "Read Device"=1432, "Read File"=1407, "ReadStatus"=1973, "Receive"=1974, "ReceiveSetup"=1975, "Recessed Box"=3601, "Recessed Circle"=3604, "Recessed Down Triangle"=3619, "Recessed Frame"=3607, "Recessed Left Triangle"=3616, "Recessed Menu Ring"=3019, "Recessed Right Triangle"=3617, "Recessed Rounded Box"=3610, "Recessed Up Triangle"=3618, "Reciprocal"=1059, "Reciprocal Of Pi"=2017, "Reciprocal Of e"=2021, "Rectangular Stop Button"=3128, "Refnum to Path"=1424, "Refnum to Session"=2306, "Register Event Callback"=2078, "Register For Events"=2065, "Register Session"=2319, "Release Notifier"=9102, "Release Queue"=9109, "Replace Array Subset"=3910, "Replace Substring"=3913, "Request Deallocation"=1610, "ResetSys"=1976, "Reshape Array"=2055, "Reverse 1D Array"=1900, "Reverse String"=1537, "Right Arrow"=3825, "Right Bow Valve"=21765, "Right Bow Valve 1"=3805, "Right Bow Valve 2"=3705, "Right Down Elbow"=3817, "Right Down Elbow 1"=3717, "Right Pump"=3719, "Right Pump 1"=3819, "Right Rect Valve"=3704, "Right Rect Valve 1"=3804, "Right Rect Valve 2"=21764, "Right Tee"=3715, "Right Tee 1"=3815, "Right Up Elbow"=3814, "Right Up Elbow 1"=3714, "Ring Constant"=2008, "Rocker"=21002, "Rotary Feeder"=3830, "Rotate"=1082, "Rotate 1D Array"=1906, "Rotate Left With Carry"=1606, "Rotate Right With Carry"=1607, "Rotate String"=1536, "Round Button"=3100, "Round LED"=3120, "Round LED 1"=21012, "Round Light"=3104, "Round Push Button"=3112, "Round Push Button 2"=3118, "Round Radio Button"=3106, "Round Stop Button"=3127, "Round To +Infinity"=1076, "Round To -Infinity"=1075, "Round To Nearest"=1055, "Rydberg Constant (/m)"=2031, "Scale By Power Of 2"=1074, "Scan From File"=2082, "Scan From String"=2080, "Scan String For Tokens"=8101, "Scan Value"=1534, "Search 1D Array"=1901, "Search and Replace String"=3914, "Search/Split String"=1538, "Secant"=1203, "Seconds To Date/Time"=1309, "Seek"=1409, "Select"=1516, "Send"=1977, "Send Notification"=9104, "SendCmds"=1978, "SendDataBytes"=1979, "SendIFC"=1980, "SendLLO"=1982, "SendList"=1981, "SendSetup"=1983, "Session to Refnum"=2307, "Set Menu Item Info"=9006, "Set Occurrence"=1702, "Set Variant Attribute"=8204, "Set Waveform Attribute"=8207, "SetRWLS"=1984, "SetTimeOut"=1985, "Sign"=1049, "Simple Horizontal Slide"=3003, "Simple Numeric"=3029, "Simple Numeric 1"=2900, "Simple String"=2115, "Simple Vertical Slide"=3002, "Sinc"=1227, "Sine"=1200, "Sine & Cosine"=1220, "Single Selection Listbox"=21200, "Size Handle"=1603, "Slide Switch"=21011, "Sort 1D Array"=1120, "Speed Of Light In Vacuum (m/sec)"=2028, "Split 1D Array"=1908, "Split Button"=21020, "Split Number"=1170, "Split Signals"=2351, "Spreadsheet String To Array"=1539, "Square Button"=3101, "Square LED"=3121, "Square LED 1"=21013, "Square Light"=3105, "Square Push Button"=3113, "Square Push Button 2"=3119, "Square Radio Button"=3107, "Square Root"=1060, "Stacked Sequence Structure"=2000, "Standard ListBox"=3202, "State Diagram"=2051, "Static VI Reference"=2084, "Stop"=1350, "Stop Button"=21230, "String Constant"=2007, "String Control"=3200, "String Control 1"=21701, "String Indicator"=3201, "String Indicator 1"=21702, "String Length"=1502, "String Subset"=1503, "String To Byte Array"=1608, "String To IP"=1711, "String To Path"=1078, "String to Tag"=1830, "Strip Path"=1420, "SubPanel"=21810, "SubPanel (Classic)"=21811, "Subtract"=1051, "Swap Bytes"=1162, "Swap Vector Element"=1912, "Swap Words"=1163, "TCP Close Connection"=1713, "TCP Create Listener"=1717, "TCP Flattened Read"=1718, "TCP Flattened Write"=1719, "TCP Flex Read"=1720, "TCP Flex Write"=1721, "TCP Network Connection Refnum"=3407, "TCP Open Connection"=1715, "TCP Read"=1716, "TCP Wait On Listener"=1712, "TCP Write"=1714, "Tab Constant"=2012, "Tab Control"=3332, "Tab Control 1"=3330, "Table"=21212, "Table 1"=3301, "Table 2"=21202, "Tag Attribute Ring"=2063, "Tag Constant"=2089, "Tag Control"=21742, "Tag Control 1"=3302, "Tag Indicator"=21743, "Tag Indicator 1"=3303, "Tag to String"=1831, "Tangent"=1202, "Tank"=3020, "Tank 1"=21006, "Temporary Directory"=1435, "TestSRQ"=1986, "TestSys"=1987, "Text & Pict Ring"=21603, "Text & Pict Ring 1"=3016, "Text Button"=21015, "Text Ring"=21601, "Text Ring 1"=3014, "Thermometer"=21007, "Thermometer 1"=3021, "Thick Chiseled Line"=3630, "Thick Line"=3629, "Thick Line with Arrow"=3631, "Thick Lowered Box"=3635, "Thin Chiseled Line"=3627, "Thin Line"=3626, "Thin Line with Arrow"=3628, "Threshold 1D Array"=1909, "Tick Count (ms)"=1300, "Time Stamp Constant"=2068, "Time Stamp Control"=5555, "Time Stamp Control 1"=21913, "Time Stamp Indicator"=5556, "Time Stamp Indicator 1"=21914, "Timed Loop"=5570, "To Byte Integer"=1140, "To Double Precision Complex"=1152, "To Double Precision Float"=1147, "To Extended Precision Complex"=1154, "To Extended Precision Float"=1149, "To Long Integer"=1142, "To Lower Case"=1189, "To More Generic Class"=8017, "To More Specific Class"=8016, "To OLE Variant"=8002, "To Quad Integer"=1155, "To Single Precision Complex"=1151, "To Single Precision Float"=1146, "To Time Stamp"=5560, "To Unsigned Byte Integer"=1143, "To Unsigned Long Integer"=1145, "To Unsigned Quad Integer"=1156, "To Unsigned Word Integer"=1144, "To Upper Case"=1188, "To Variant"=8201, "To Word Integer"=1141, "Traditional DAQ Channel"=21733, "Traditional DAQ Channel 1"=3320, "Traditional DAQ Channel Constant"=2085, "Transpose 2D Array"=1902, "Tree"=21793, "Trigger"=1988, "TriggerList"=1989, "Two Button Dialog"=1341, "Type Cast"=1166, "Type and Creator"=1434, "UDP Close"=1726, "UDP Multicast Open"=1727, "UDP Network Connection Refnum"=3418, "UDP Open"=1723, "UDP Read"=1724, "UDP Write"=1725, "Unbundle"=2048, "Unbundle By Name"=2058, "Unflatten From String"=1161, "Unflatten From XML"=8401, "Uniform Dbl Waveform"=3312, "Uniform Int16 Waveform"=3313, "Unregister For Events"=2076, "Unregister Session"=2320, "Up Arrow"=3823, "Up Bow Valve"=3703, "Up Bow Valve 1"=3803, "Up Bow Valve 2"=21763, "Up Rect Valve"=3702, "Up Rect Valve 1"=21762, "Up Rect Valve 2"=3802, "Up Tee"=3712, "Up Tee 1"=3812, "User Item"=3506, "VI Library"=1425, "VI Refnum"=3422, "VISA Assert Interrupt Signal"=2309, "VISA Assert Trigger"=1929, "VISA Assert Utility Signal"=2310, "VISA Clear"=1927, "VISA Close"=1922, "VISA Disable Event"=1940, "VISA Discard Events"=1941, "VISA Enable Event"=1942, "VISA Find Resource"=1923, "VISA Flush I/O Buffer"=2302, "VISA GPIB Command"=2315, "VISA GPIB Control ATN"=2316, "VISA GPIB Control REN"=2304, "VISA GPIB Pass Control"=2317, "VISA GPIB Send IFC"=2318, "VISA In 16"=1930, "VISA In 32"=1944, "VISA In 8"=1936, "VISA Lock"=1993, "VISA Map Address"=1932, "VISA Map Trigger"=2311, "VISA Memory Allocation"=1997, "VISA Memory Free"=1998, "VISA Move"=2303, "VISA Move In 16"=1948, "VISA Move In 32"=1991, "VISA Move In 8"=1946, "VISA Move Out 16"=1949, "VISA Move Out 32"=1992, "VISA Move Out 8"=1947, "VISA Open"=2308, "VISA Out 16"=1931, "VISA Out 32"=1945, "VISA Out 8"=1937, "VISA Peek 16"=1934, "VISA Peek 32"=1995, "VISA Peek 8"=1938, "VISA Poke 16"=1935, "VISA Poke 32"=1996, "VISA Poke 8"=1939, "VISA Read"=1925, "VISA Read STB"=1928, "VISA Read To File"=2313, "VISA Refnum to Session"=2300, "VISA Resource Name"=21737, "VISA Resource Name Constant"=3421, "VISA Set I/O Buffer Size"=2301, "VISA Status Description"=1924, "VISA USB Control In"=2086, "VISA USB Control Out"=2087, "VISA Unlock"=1994, "VISA Unmap Address"=1933, "VISA Unmap Trigger"=2312, "VISA VXI Cmd or Query"=2305, "VISA Wait on Event"=1943, "VISA Write"=1926, "VISA Write From File"=2314, "VISA resource name"=3409, "Variant"=3310, "Variant To Data"=8003, "Variant To Flattened String"=8203, "Vert Line"=3822, "Vert Pipe"=3816, "Vert Pipe 1"=3716, "Vert Rocker"=21740, "Vertical Fill Slide"=21014, "Vertical Fill Slide 1"=3009, "Vertical Graduated Bar"=21107, "Vertical Pointer Slide"=21017, "Vertical Pointer Slide 1"=3007, "Vertical Progress Bar"=21104, "Vertical Slide"=3004, "Vertical Slide Switch"=21741, "Vertical Slide Switch 1"=3115, "Vertical Smooth Box"=3634, "Vertical Switch"=3109, "Vertical Toggle Switch"=21005, "Vertical Toggle Switch 1"=3111, "Volume Info"=1414, "Wait (ms)"=1302, "Wait For Activity"=1722, "Wait For Front Panel Activity"=1328, "Wait Until Next ms Multiple"=1327, "Wait for GPIB RQS"=1952, "Wait on Notification"=9105, "Wait on Notification from Multiple"=9106, "Wait on Occurrence"=1701, "WaitSRQ"=1990, "Waveform Chart"=21010, "Waveform Chart 1"=3501, "Waveform Chart 2"=21717, "Waveform Graph"=21703, "Waveform Graph 1"=3504, "While Loop"=2003, "While Loop 1"=2352, "White Space?"=1125, "Write Device"=1431, "Write File"=1408, "XY Graph"=3500, "XY Graph 1"=21716] ("New VI Object Style")
                  n98 = property class="VI"(reference=w267, error in=w264) -> (reference out=w262:refnum<vi>, error out=w263:errorcluster, "Panel"=w256:refnum<vi>)
                  n99 = New VI Object(vi object class=w268, owner refnum=w256, style=w269, position/next to=T2 {"Horizontal"=300, "Vertical"=300} ("relative position/next to refnum"), 8:w263) -> (object refnum=w259:refnum<vi>, 0:w265:errorcluster)  [unwired: 3 in]
                  n100 = invoke class="VI" method="Save.Instrument"(reference=w262, error in=w265) -> (reference out=w261:refnum<vi>, error out=w260:errorcluster)  [unwired: 4 in, 4 out]
                  n101 = invoke class="Str" method="Delete"(reference=w259, error in=w260) -> (reference out=w257:refnum<vi>, error out=w258:errorcluster)  [unwired: 1 in, 1 out]
                  n102 = invoke class="VI" method="Save.Instrument"(reference=w261, error in=w258) -> (error out=w255:errorcluster)  [unwired: 4 in, 5 out]
                  n103 = Close Reference(reference=w257, error in (no error)=w255) -> ()  [unwired: 1 out]
                  n104 = Close Reference(reference=w256, error in (no error)=w255) -> ()  [unwired: 1 out]
                }
              }
            }
          }
          frame "RenameClassControlsIfNeeded" {
            n105 = disable-structure shown="Enabled" {
              disable-tunnel: w274 -> [w280 w317]
              disable-tunnel: [w279 w318] -> w273
              disable-tunnel: w272 -> [w277 w319]
              disable-tunnel: w270 -> [_ _]
              frame Disabled {
                n106 = Unbundle By Name(w280) -> ("VIRefs"=w278:refnum<vi>[], "OrgClassName"=w276:string, "NewClassName"=w275:string)
                n107 = for {
                  shift-right: [w281] -> w279
                  shift-left: w277 -> [w289]
                  tunnel: w278 -> [w290] mode=indexing
                  tunnel: w276 -> [w285]
                  tunnel: w275 -> [w284]
                  n108 = property class="VI"(reference=w290, error in=w289) -> (error out=w288:errorcluster, "Panel"=w291:refnum<vi>)  [unwired: 1 out]
                  n109 = property class="Pnl"(reference=w291, error in=w288) -> (reference out=w282:refnum<vi>, error out=w286:errorcluster, "Controls[]"=w287:refnum<vi>[])
                  n110 = for {
                    tunnel: w287 -> [w301] mode=indexing
                    shift-right: [w292] -> w283
                    shift-left: w286 -> [w298]
                    tunnel: w285 -> [w297]
                    tunnel: w284 -> [w296]
                    n111 = property class="Ctl" props=["ClassName", "Label", "Text", "Typedef Path"](reference=w301, error in=w298) -> (reference out=w293:refnum<vi>, error out=w295:errorcluster, "ClassName"=w300:string, "Label.Text"=w299:string)  [unwired: 1 out]
                    n112 = case shown="\"LabVIEWClassControl\"" w300 {
                      tunnel: w299 -> [_ w309]
                      tunnel: w293 -> [_ w310]
                      tunnel: w297 -> [_ w306]
                      tunnel: w296 -> [_ w305]
                      tunnel: w295 -> [w302 w304]
                      tunnel: [w302 w303] -> w294
                      frame Default {
                      }
                      frame "LabVIEWClassControl" {
                        n113 = Search and Replace String(input string=w309, search string=w306, replace string=w305) -> (result string=w308:string, number of replacements=w307:i32)  [unwired: 5 in, 2 out]
                        n114 = case shown="0, Default" w307 {
                          tunnel: w310 -> [_ w315]
                          tunnel: w308 -> [_ w314]
                          tunnel: w304 -> [w311 w313]
                          tunnel: [w311 w312] -> w303
                          frame 0, Default {
                          }
                          frame 1.. {
                            n115 = property class="Ctl"(reference=w315, error in=w313, "Label.Text"=w314) -> (error out=w312:errorcluster)  [unwired: 1 out]
                          }
                        }
                      }
                    }
                    n116 = Close Reference(reference=w293, error in (no error)=w294) -> (error out=w292:errorcluster)
                  }
                  n117 = Close Reference(reference=w282, error in (no error)=w283) -> (error out=w281:errorcluster)
                }
              }
              frame Enabled {
                n118 = Unbundle By Name(w317) -> ("NewClass"=w316:refnum<vi>)
                n119 = call <resource>:"Scripting_RenameClassControlsOfClass.vi"("error in (no error)"=w319, "LVClassLibrary in"=w316) -> ("error out"=w318:errorcluster)  [unwired: 9 in]
              }
            }
          }
          frame "CloseRefs", "Error", Default {
            n120 = Unbundle By Name(w328) -> ("VIRefs"=w322:refnum<vi>[], "NewClass"=w342:refnum<vi>, "ProjectItemToAddTo"=w339:refnum<vi>, "Application"=w325:refnum<vi>)
            n121 = Close Reference(reference=w322, error in (no error)=w321) -> (error out=w320:errorcluster)
            n122 = call <resource>:"GDSLvClass_SaveEverythingInClass.vi"("ClassRefIn"=w342, "ForceResaving(False)"=TRUE, "error in"=w320) -> ("ClassRefOut"=w331:refnum<vi>, "error out"=w332:errorcluster)  [unwired: 15 in]
            n123 = property class="LVClassLibrary"(reference=w331, error in=w332) -> (reference out=w330:refnum<vi>, error out=w329:errorcluster, "Path"=w326:path)
            n124 = Bundle By Name(cluster=w328, "Path"=w326) -> (w327:T1)
            n125 = Close Reference(reference=w330, error in (no error)=w329) -> (error out=w340:errorcluster)
            n126 = property class="ProjectItem"(reference=w339, error in=w340) -> (reference out=w338:refnum<vi>, error out=w336:errorcluster, "Project"=w337:refnum<vi>)
            n127 = invoke class="Project" method="Save"(reference=w337, error in=w336) -> (reference out=w334:refnum<vi>, error out=w335:errorcluster)  [unwired: 2 in, 2 out]
            n128 = Close Reference(reference=w338, error in (no error)=w335) -> (error out=w333:errorcluster)
            n129 = Close Reference(reference=w334, error in (no error)=w333) -> (error out=w324:errorcluster)
            n130 = Close Reference(reference=w325, error in (no error)=w324) -> (error out=w323:errorcluster)
          }
          frame "TempFix" {
            n131 = case shown="True" FALSE {
              tunnel: w347 -> [_ w353]
              tunnel: w346 -> [w349 w352]
              tunnel: [w349 w351] -> w345
              frame False {
              }
              frame True {
                n132 = case shown="False" TRUE {
                  tunnel: w353 -> [w355 w373]
                  tunnel: w352 -> [w367 w369]
                  tunnel: [w367 w369] -> w351
                  frame False {
                    (unwired) TRUE ("ForceResaving(False)")
                    n133 = Unbundle By Name(w355) -> ("NewClass"=w354:refnum<vi>)
                    n134 = property class="LVClassLibrary"(reference=w354) -> (reference out=w360:refnum<vi>, error out=w361:errorcluster, "Parent"=w366:refnum<vi>)  [unwired: 1 in]
                    n135 = property class="LVClassLibrary"(reference=w360, error in=w361, "Parent"=refnum<k0> refnum) -> (reference out=w357:refnum<vi>, error out=w358:errorcluster)
                    n136 = call <resource>:"GDSLvClass_SaveEverythingInClass.vi"("ClassRefIn"=w357, "error in"=w358) -> ("ClassRefOut"=w359:refnum<vi>, "error out"=w362:errorcluster)  [unwired: 16 in]
                    n137 = property class="LVClassLibrary"(reference=w359, error in=w362, "Parent"=w366) -> (reference out=w363:refnum<vi>, error out=w364:errorcluster)
                    n138 = call <resource>:"GDSLvClass_SaveEverythingInClass.vi"("ClassRefIn"=w363, "error in"=w364) -> ("error out"=w365:errorcluster)  [unwired: 16 in, 1 out]
                    n139 = Close Reference(reference=w366, error in (no error)=w365) -> ()  [unwired: 1 out]
                  }
                  frame True {
                    w368 = TRUE ("ExcludeDependencies")
                    n140 = Unbundle By Name(w373) -> ("NewClass"=w371:refnum<vi>)
                    n141 = invoke class="LVClassLibrary" method="Get All Descendents"(reference=w371, "Type"="VI", "Exclude Dependencies"=w368, "ExcludeBuilds"=w368) -> ("All Descendents"=w370:refnum<vi>[])  [unwired: 3 in, 6 out]
                    n142 = for {
                      tunnel: w370 -> [w376] mode=indexing
                      n143 = property class="ProjectItem"(reference=w376) -> ("Reference"=w375:refnum<vi>)  [unwired: 1 in, 2 out]
                      n144 = Not A Number/Path/Refnum?(number/path/refnum=w375) -> ()  [unwired: 1 out]
                      n145 = case shown="False" TRUE {
                        tunnel: w375 -> [w380 _]
                        frame False {
                          n146 = property class="VI"(reference=w380) -> (reference out=w378:refnum<vi>, "VIType"=w379:T4, "Panel"=w377:refnum<vi>)  [unwired: 1 in, 1 out]
                          n147 = case shown="Default" w379 {
                            tunnel: w378 -> [w383 _]
                            tunnel: w377 -> [_ _]
                            frame Default {
                              n148 = invoke class="VI" method="Save.Instrument"(reference=w383) -> (reference out=w382:refnum<vi>, error out=w381:errorcluster)  [unwired: 5 in, 4 out]
                              n149 = invoke class="VI" method="Revert VI"(reference=w382, error in=w381) -> ()  [unwired: 1 in, 3 out]
                            }
                            frame "Control VI" {
                            }
                          }
                        }
                        frame True {
                        }
                      }
                    }
                  }
                }
              }
            }
          }
        }
        n150 = Equal?(x=w25, y="Exit") -> (x = y?=w28:bool)
        n151 = Select(t="Error", s=w24, f=w25) -> (s? t:f=w29:string)
      }
      n152 = Unbundle By Name(w11) -> ("Path"=w10:path)
    }
    frame Error {
    }
  }
  "ClassWriterNative.lvclass" <- w6
  "error out" <- w8
  "NewClassPathOut(Might Be Modified)" <- w1
